vi "PruebaCalibration.vi"() -> ()   [LabVIEW 2014, in "MSX-E3711_dll.lvlib"]
uses:
  MSX-E3711_dll.lvlib
  Typedef/Connection Data.ctl
  E:/Repositorio Magnis/INF002/v0/Modules/HAL/Drivers/Sync/ADDI-DATA MSX-E3711/API/MSXE371x.dll
  MSXE371x.dll
  E:/Repositorio Magnis/INF002/v0/Modules/HAL/Drivers/Sync/ADDI-DATA MSX-E3711/API/MXCommon.dll
  MXCommon.dll
  Typedef/Calibration Data.ctl
panel:
  out "Cluster Calibration":T1
  in  "Connection Data In":T2
  in  "stop":bool
  # "Information"
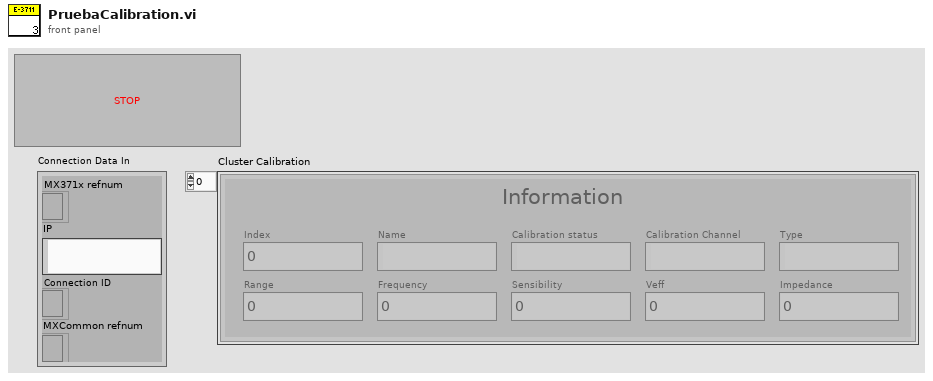
[diagram p1: front panel]
types:
  T1 = typedef "MSX-E3711_dll.lvlib/Calibration Data.ctl" = cluster{"Calibration status":string, "Name":string, "Index":u64, "Range":dbl, "Sensibility":dbl, "Veff":dbl, "Frequency":u64, "Impedance":u64, "Type":string, "Calibration Channel":string}[]
  T2 = typedef "MSX-E3711_dll.lvlib/Connection Data.ctl" = cluster{"MX371x refnum":refnum<k24>, "IP":string, "Connection ID ":refnum<k5>, "MXCommon refnum":refnum<k24>}
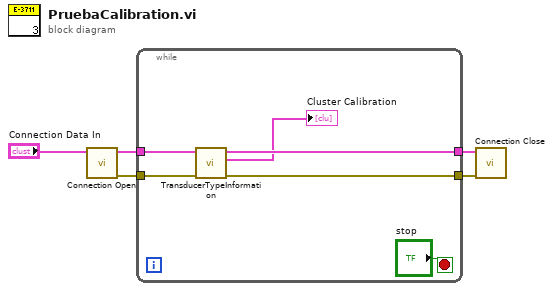
[diagram p0: block diagram]
diagram:
  n1 = call "Connection Open.vi"("Connection Data In"="Connection Data In") -> ("error out"=w3:errorcluster, "Connection Data Out"=w5:T2)  [unwired: 9 in]
  n2 = while {
    tunnel: w5 -> [w11]
    tunnel: [w10] -> w4
    tunnel: w3 -> [w9]
    tunnel: [w8] -> w2
    stop <- "stop" stop-if-true
    n3 = call "TransducerTypeInformation.vi"("error in (no error)"=w9, "Connection Data In"=w11) -> ("error out"=w8:errorcluster, "Cluster Calibration"=→"Cluster Calibration":T1, "Connection Data Out"=w10:T2)  [unwired: 7 in]
  }
  n4 = call "Connection Close.vi"("error in (no error)"=w2, "Connection Data In"=w4) -> ()  [unwired: 8 in, 2 out]
